vi "Write Cycle_.vi"(8 "error in (no error)":errorcluster, 10 "Cycle?":bool, 11 "Toggle Filter Cycle MSG in":refnum<class "Toggle Filter Cycle MSG.lvclass">) -> (0 "error out":errorcluster, 3 "Toggle Filter Cycle MSG out":refnum<class "Toggle Filter Cycle MSG.lvclass">)   [LabVIEW 2014, in "Controller.lvlib" / "Toggle Filter Cycle MSG.lvclass"]
uses:
  Toggle Filter Cycle MSG.lvclass
  Toggle Filter Cycle MSG.lvclass/Toggle Filter Cycle MSG.ctl
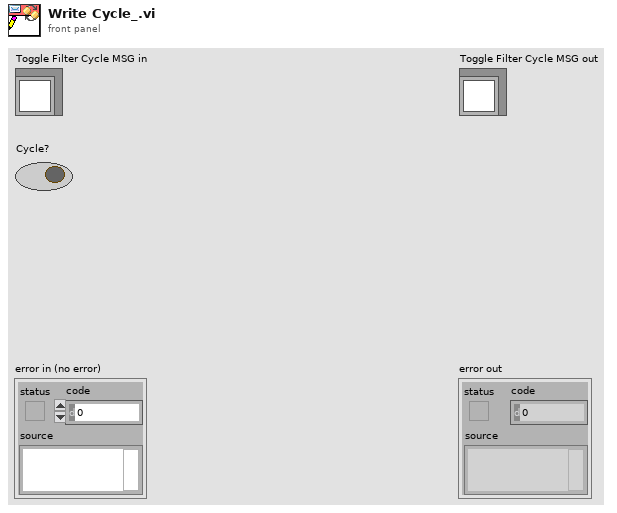
[diagram p1: front panel]
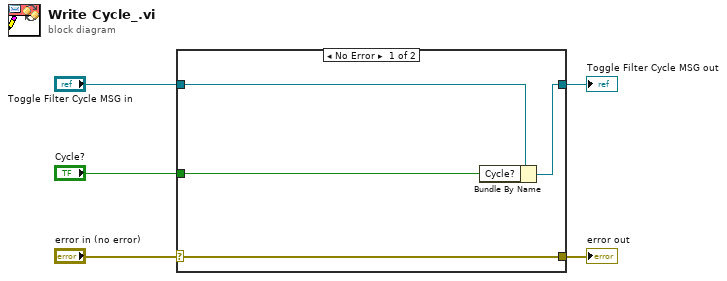
[diagram p0: block diagram]
diagram:
  n1 = case shown="No Error" "error in (no error)" {
    selector: "error in (no error)" -> [w9 w10]
    tunnel: [w9 w10] -> w4
    tunnel: [w7 w11] -> w2
    tunnel: "Toggle Filter Cycle MSG in" -> [w8 w11]
    tunnel: "Cycle?" -> [w6 _]
    frame No Error {
      n2 = Bundle By Name(cluster=w8, "Cycle?"=w6) -> (w7:refnum<class "Toggle Filter Cycle MSG.lvclass">)
    }
    frame Error {
    }
  }
  "error out" <- w4
  "Toggle Filter Cycle MSG out" <- w2
